vi "Configure Multiple Points.vi"(8 "error in":errorcluster, 9 "Enable Burst Action (F: Disable)":bool, 10 "Sample Count (1)":i32=1 min=1 max=8000 step=1, 11 "VISA resource name":refnum<visa-resource-name>) -> (0 "error out":errorcluster, 3 "VISA resource name out":refnum<visa-resource-name>)   [LabVIEW 2017, in "ADCMT 6240.lvlib"]
doc: "Configures multiple measurement points"
uses:
  ADCMT 6240.lvlib
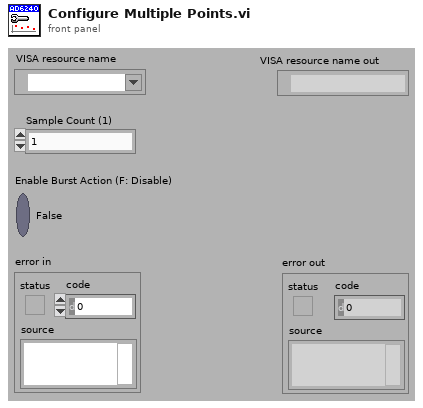
[diagram p1: front panel]
types:
  T1 = typedef "ADCMT 6240.lvlib/Extended User Data.ctl" = cluster{"Trigger Mode":u16, "Output Mode":u16, "Sample Count":i32, "Model":u16}
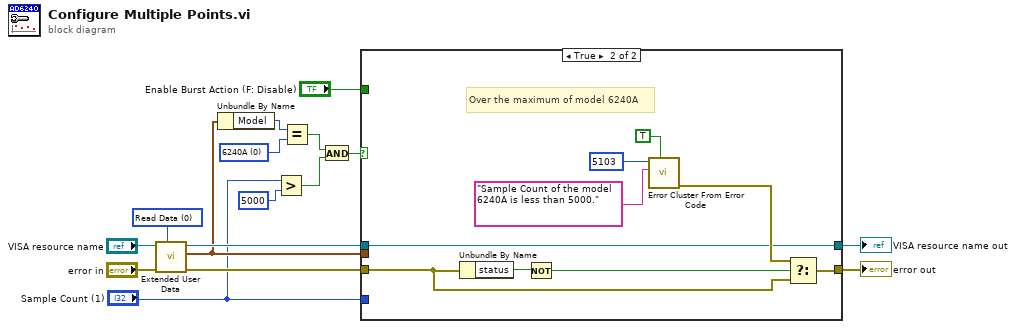
[diagram p0: block diagram]
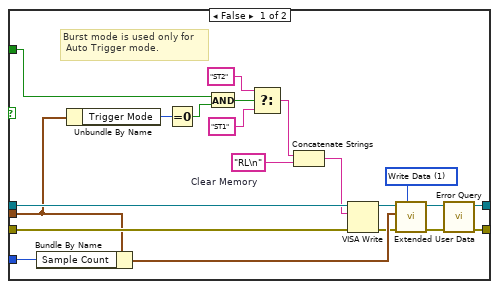
[diagram p2: hidden frame]
diagram:
  w8 = u16 0 items=["6240A", "6240B"] ("Model")
  w14 = u16 0 items=["Read Data", "Write Data", "Dispose of Data"] ("Action")
  n1 = call "Extended User Data.vi"("Action"=w14, "Error In (no error)"="error in", "VISA resource name in"="VISA resource name") -> ("Error Out"=w11:errorcluster, "User Data Out"=w9:T1, "VISA resource name out"=w10:refnum<visa-resource-name>)  [unwired: 6 in]
  n2 = Unbundle By Name(w9) -> ("Model"=w7:u16)
  n3 = Greater?(x="Sample Count (1)", y=5000) -> (0:w3:bool)
  n4 = Equal?(x=w7, y=w8) -> (x = y?=w4:bool)
  n5 = And(x=w4, y=w3) -> (x .and. y?=w2:bool)
  n6 = case shown="True" w2 {
    tunnel: [w37 w39] -> w16
    tunnel: [w36 w41] -> w15
    tunnel: w11 -> [w25 w40]
    tunnel: w10 -> [w24 w41]
    tunnel: w9 -> [w19 _]
    tunnel: "Sample Count (1)" -> [w18 _]
    tunnel: "Enable Burst Action (F: Disable)" -> [w17 _]
    frame False {
      w31 = "RL\n"  # Clear Memory
      w35 = u16 1 items=["Read Data", "Write Data", "Dispose of Data"] ("Action")
      # "Burst mode is used only for\n Auto Trigger mode."
      n7 = Bundle By Name(cluster=w19, "Sample Count"=w18) -> (w30:T1)
      n8 = Unbundle By Name(w19) -> ("Trigger Mode"=w33:u16)
      n9 = Equal To 0?(x=w33) -> (x = 0?=w21:bool)
      n10 = And(x=w17, y=w21) -> (x .and. y?=w22:bool)
      n11 = Select(t="ST2", s=w22, f="ST1") -> (s? t:f=w23:string)
      n12 = Concatenate Strings(w23, w31) -> (w20:string)
      n13 = VISA Write ("VISA書き込み")(VISA resource name=w24, write buffer=w20, error in (no error)=w25) -> (VISA resource name out=w29:refnum<visa-resource-name>, error out=w26:errorcluster)  [unwired: 1 out]
      n14 = call "Extended User Data.vi"("Action"=w35, "Error In (no error)"=w26, "User Data In"=w30, "VISA resource name in"=w29) -> ("Error Out"=w27:errorcluster, "VISA resource name out"=w28:refnum<visa-resource-name>)  [unwired: 5 in, 1 out]
      n15 = call "Error Query.vi"("error in (no error)"=w27, "VISA resource name"=w28) -> ("error out"=w37:errorcluster, "VISA resource name out"=w36:refnum<visa-resource-name>)  [unwired: 6 in, 2 out]
    }
    frame True {
      # "Over the maximum of model 6240A"
      n16 = Unbundle By Name(w40) -> ("status"=w44:bool)
      n17 = Not(x=w44) -> (.not. x?=w43:bool)
      n18 = call <vilib>:"Error Cluster From Error Code.vi"("show call chain? (False)"=TRUE, "error message (\"\")"="Sample Count of the model 6240A is less than 5000." ("Source (VI Name)"), "error code (0)"=5103 ("Code")) -> ("error out"=w42:errorcluster)  [unwired: 6 in]
      n19 = Select(t=w42, s=w43, f=w40) -> (s? t:f=w39:errorcluster)
    }
  }
  "VISA resource name out" <- w15
  "error out" <- w16
